vi "Get-Set Inspection Limits.vi"(6 "wait for reply (T)":bool=TRUE, 8 "error in (no error)":errorcluster, 10 "Inspection Limits":T2={"MaxSamples"=50800, "PosToStartScan"=50800, "PosToEndScan"=0, "ScanLength"=50800}, 11 "Set":bool) -> (0 "error out":errorcluster, 1 "timed out?":bool, 2 "Reply Payload":T1={"Inspection Limits"={"MaxSamples"=50800, "PosToStartScan"=50800, "PosToEndScan"=0, "ScanLength"=50800}, "Get-Set Inspection Limits_error"={"status"=FALSE, "code"=0, "source"=""}})   [LabVIEW 2015, in "Tool Module.lvlib"]
doc: "Get or Set the Inspection Limits. These are local parameters for the Tool Module operation (not in the tool).\n_____\nCreated using Delacor QMH Event Scripter 4.2.1.88."
uses:
  Tool Module.lvlib
  Support/_Inspection Limits cluster--typedef.ctl
  Get-Set Inspection Limits (Reply Payload)--cluster.ctl
  Get-Set Inspection Limits Argument--cluster.ctl
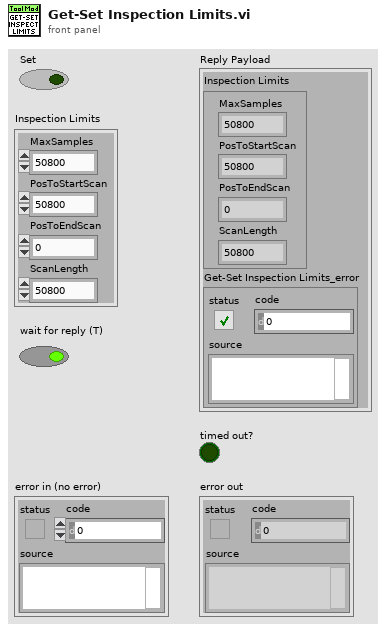
[diagram p1: front panel]
types:
  T1 = typedef "Tool Module.lvlib/Get-Set Inspection Limits (Reply Payload)--cluster.ctl" = cluster{"Inspection Limits":T2, "Get-Set Inspection Limits_error":errorcluster}
  T2 = typedef "Tool Module.lvlib/_Inspection Limits cluster--typedef.ctl" = cluster{"MaxSamples":i32, "PosToStartScan":i32, "PosToEndScan":i32, "ScanLength":i32}
  T3 = typedef "Tool Module.lvlib/Get-Set Inspection Limits Argument--cluster.ctl" = cluster{"Set":bool, "Inspection Limits":T2, "Wait Notifier":refnum<notifier>, "wait for reply":bool}
  T4 = typedef "Tool Module.lvlib/Request Events--cluster.ctl" = cluster{"Stop Module":refnum<user-event>, "Show Panel":refnum<user-event>, "Hide Panel":refnum<user-event>, "Get Module Execution Status":refnum<user-event>, "Show Diagram":refnum<user-event>, "GOTO":refnum<user-event>, "Start Inspect":refnum<user-event>, "CONNECT":refnum<user-event>, "Get All Inspect Data":refnum<user-event>, "Start Data Monitor":refnum<user-event>, "Get FPGA Setup Params":refnum<user-event>, "Set FPGA Setup Params":refnum<user-event>, "Set Tool Config":refnum<user-event>, "Get Tool Config":refnum<user-event>, "Set Integration Count":refnum<user-event>, "Set Laser Params":refnum<user-event>, "Get Mtrl Ctrl Reg":refnum<user-event>, "Commit Ctrl Reg":refnum<user-event>, "Set Event Logger":refnum<user-event>, "Write to File":refnum<user-event>, "Read from File":refnum<user-event>, "Set Device Temp Thresholds":refnum<user-event>, "Get Cycle Count":refnum<user-event>, "Return FPGA Setup Data":refnum<user-event>, "Update FPGA Setup Data":refnum<user-event>, "Setup Timer":refnum<user-event>, "Tool Status Reader Cmd":refnum<user-event>, "Stop Helper Loops":refnum<user-event>, "Timer Complete":refnum<user-event>, "Enable Receive Stream":refnum<user-event>, "Get-Set Inspection Limits":refnum<user-event>}
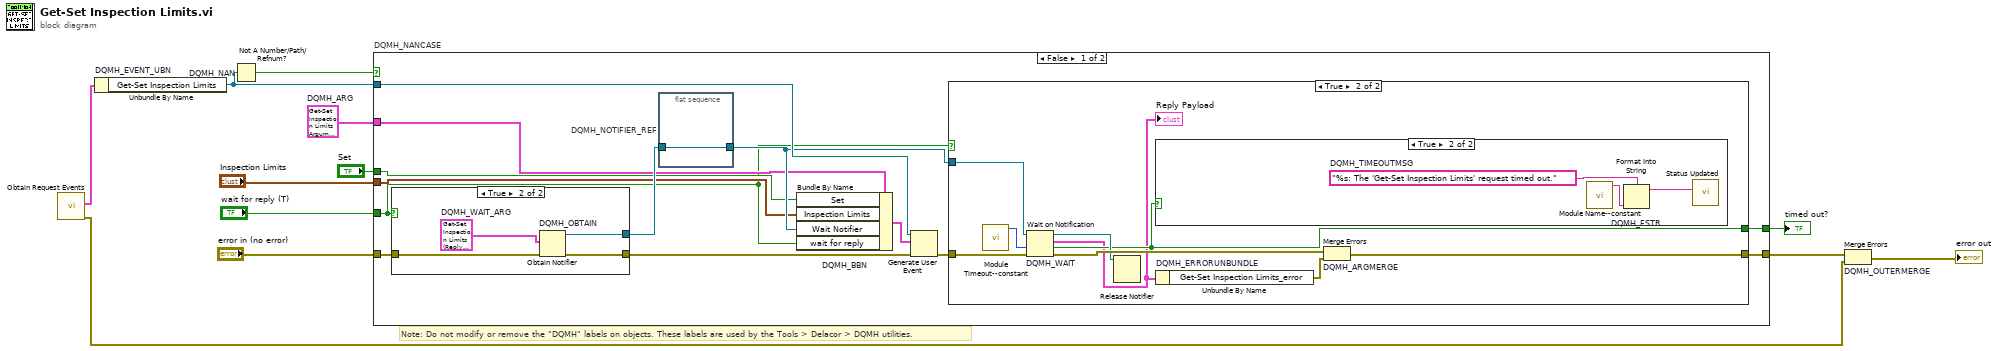
[diagram p0: block diagram]
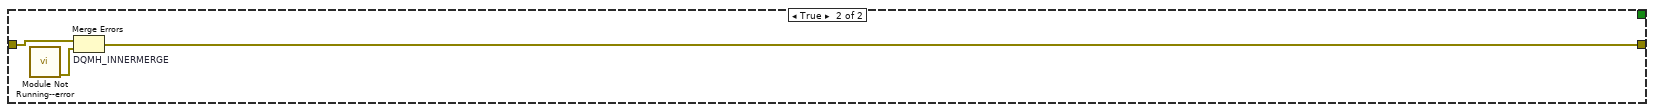
[diagram p5: hidden frame]
diagram:
  w6 = T3 {"Set"=FALSE, "Inspection Limits"={"MaxSamples"=50800, "PosToStartScan"=50800, "PosToEndScan"=0, "ScanLength"=50800}, "Wait Notifier"=refnum, "wait for reply"=FALSE}  # DQMH_ARG
  # "Note: Do not modify or remove the \"DQMH\" labels on objects. These labels are used by the Tools > Delacor > DQMH utilities."
  n1 = call "Obtain Request Events.vi"() -> ("error out"=w2:errorcluster, "Tool Module Request Events"=w1:T4)  [unwired: 10 in]
  n2 = Unbundle By Name "DQMH_EVENT_UBN"(w1) -> ("Get-Set Inspection Limits"=w10:refnum<user-event>)
  n3 = Not A Number/Path/Refnum? "DQMH_NAN"(number/path/refnum=w10) -> (NaN/Path/Refnum?=w9:bool)
  n4 = case "DQMH_NANCASE" shown="False" w9 {
    tunnel: "error in (no error)" -> [w25 w47]
    tunnel: w10 -> [w23 _]
    tunnel: [w20 w46] -> w7
    tunnel: [w21 _] -> w8
    tunnel: w6 -> [w16 _]
    tunnel: "Set" -> [w15 _]
    tunnel: "Inspection Limits" -> [w14 _]
    tunnel: "wait for reply (T)" -> [w13 _]
    frame False {
      n5 = case shown="True" w13 {
        tunnel: w25 -> [w40 w44]
        tunnel: [w40 w43] -> w22
        tunnel: [_ w41] -> w18
        frame False {
        }
        frame True {
          w42 = T1 {"Inspection Limits"={"MaxSamples"=50800, "PosToStartScan"=50800, "PosToEndScan"=0, "ScanLength"=50800}, "Get-Set Inspection Limits_error"={"status"=FALSE, "code"=0, "source"=""}}  # DQMH_WAIT_ARG
          n6 = Obtain Notifier "DQMH_OBTAIN"(notification data type=w42, error in (no error)=w44) -> (notifier out=w41:refnum<notifier>, error out=w43:errorcluster)  [unwired: 2 in, 1 out]
        }
      }
      n7 = flat-sequence "DQMH_NOTIFIER_REF" {
        tunnel: w18 -> [w26]
        tunnel: [w26] -> w17
        frame #0 {
        }
      }
      n8 = Bundle By Name "DQMH_BBN"(cluster=w16, "Set"=w15, "Inspection Limits"=w14, "Wait Notifier"=w17, "wait for reply"=w13) -> (w19:T3)
      n9 = Generate User Event(user event=w23, event data cluster=w19, error in=w22) -> (error out=w24:errorcluster)  [unwired: 1 in, 1 out]
      n10 = case shown="True" w13 {
        tunnel: w24 -> [w27 w36]
        tunnel: w17 -> [_ w34]
        tunnel: [_ w32] -> w21
        tunnel: [w27 w31] -> w20
        frame False {
        }
        frame True {
          n11 = call "Module Timeout--constant.vi"() -> ("Module Timeout"=w28:i32)  [unwired: 11 in]
          n12 = Wait on Notification "DQMH_WAIT"(notifier=w34, timeout in ms (-1)=w28, error in (no error)=w36) -> (notifier out=w33:refnum<notifier>, notification=w29:T1, timed out?=w32:bool, error out=w35:errorcluster)  [unwired: 1 in]
          "Reply Payload" <- w29
          n13 = Release Notifier(notifier=w33) -> ()  [unwired: 2 in, 3 out]
          n14 = case shown="True" w32 {
            frame False {
            }
            frame True {
              w39 = "%s: The 'Get-Set Inspection Limits' request timed out."  # DQMH_TIMEOUTMSG
              n15 = call "Module Name--constant.vi"() -> ("Module Name"=w38:string)  [unwired: 11 in]
              n16 = Format Into String "DQMH_FSTR"(format string=w39, w38) -> (resulting string=w37:string)  [unwired: 2 in, 1 out]
              n17 = call "Status Updated.vi"("Status"=w37) -> ()  [unwired: 10 in, 1 out]
            }
          }
          n18 = Unbundle By Name "DQMH_ERRORUNBUNDLE"(w29) -> ("Get-Set Inspection Limits_error"=w30:errorcluster)
          n19 = Merge Errors "DQMH_ARGMERGE"(w35, w30) -> (w31:errorcluster)
        }
      }
    }
    frame True {
      n20 = call "Module Not Running--error.vi"() -> ("error out"=w45:errorcluster)  [unwired: 11 in]
      n21 = Merge Errors "DQMH_INNERMERGE"(w47, w45) -> (w46:errorcluster)
    }
  }
  "timed out?" <- w8
  n22 = Merge Errors "DQMH_OUTERMERGE"(w7, w2) -> (→"error out":errorcluster)
